vi "reset_q.vi"(4 "discountfactor":dbl, 5 "learningrate":dbl, 6 "new state":dbl, 7 "Numeric":i32, 9 "reward":dbl, 10 "state":dbl, 11 "Q in":dbl[][](array[numeric])) -> (3 "Q out":dbl[][](array[numeric]))   [LabVIEW 2022 SP3]
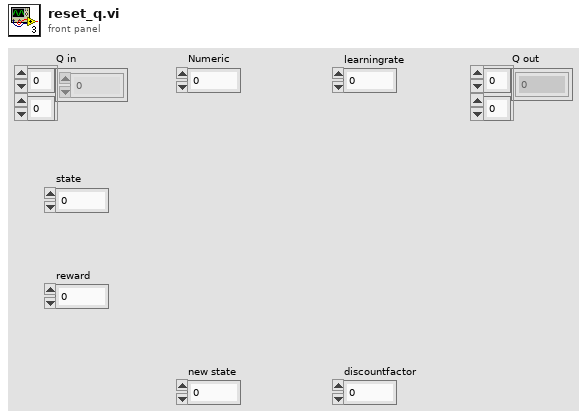
[diagram p1: front panel]
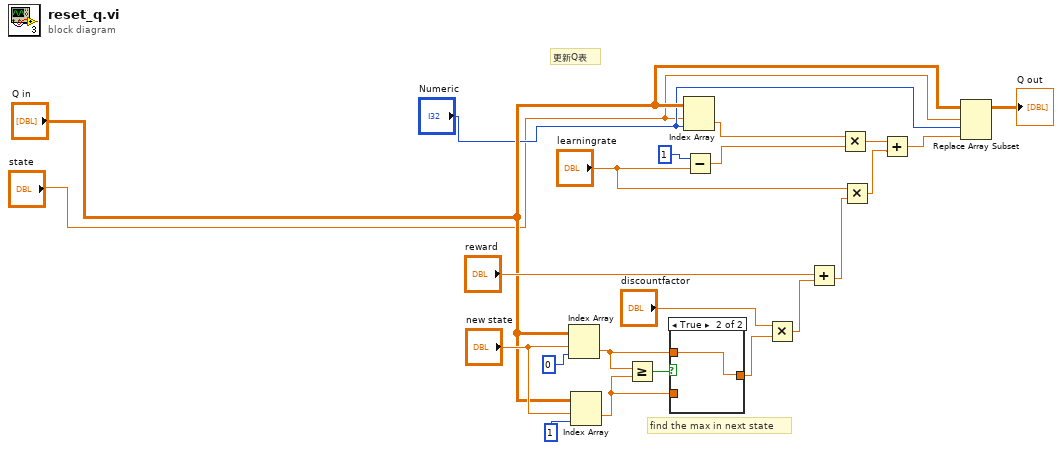
[diagram p0: block diagram]
diagram:
  # "find the max in next state"
  # "更新Q表"
  n1 = Index Array(array="Q in", index (row)="new state", index (col)=0) -> (element=w11:dbl)
  n2 = Index Array(array="Q in", index (row)="new state", index (col)=1) -> (element=w12:dbl)
  n3 = Greater Or Equal?(x=w11, y=w12) -> (x >= y?=w6:bool)
  n4 = case shown="True" w6 {
    tunnel: [w23 w24] -> w14
    tunnel: w11 -> [_ w24]
    tunnel: w12 -> [w23 _]
    frame False {
    }
    frame True {
    }
  }
  n5 = Index Array(array="Q in", index (row)="state", index (col)="Numeric") -> (element=w3:dbl)
  n6 = Subtract(x=1, y="learningrate") -> (x-y=w2:dbl)
  n7 = Multiply(x="discountfactor", y=w14) -> (x*y=w15:dbl)
  n8 = Add(x="reward", y=w15) -> (x+y=w22:dbl)
  n9 = Multiply(x=w3, y=w2) -> (x*y=w18:dbl)
  n10 = Multiply(x="learningrate", y=w22) -> (x*y=w19:dbl)
  n11 = Add(x=w18, y=w19) -> (x+y=w20:dbl)
  n12 = Replace Array Subset(array="Q in", new element=w20, index (row)="state", index (col)="Numeric") -> (→"Q out":dbl[][])
